vi "Dig a Grave - Complex.vi"() -> ()   [LabVIEW 2017]
doc: "A demonstration of digging graves for slightly more complex legacy code to be refactored. This includes step-by-step instructions for creating grave sin one of two methods: shortcut menu plugin or Quick Drop shortcut plugin. A \"grave\" is a Diagram Disable Structure with a \"Corpse\" disabled frame for the legacy code and a \"Spirit\" enabled frame with a copy of the legacy code to safely refactor."
panel:
  in  "Input":timestamp=timestamp(3614009430.8933406 s since 1904-01-01)
  in  "Stop":bool
  # "Overview: Demonstrates digging a grave for slightly more comple code that needs to be refactored\nInstructions:\n1. Run the VI\n2. Select a time and date using the Input control\n3. Observe the behavior of the VI. Does a notification dialog ever appear?\n4. Switch to the block diagram and follow the instructions there to refactor the code"
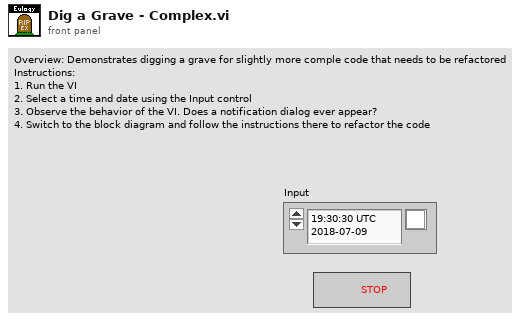
[diagram p1: front panel]
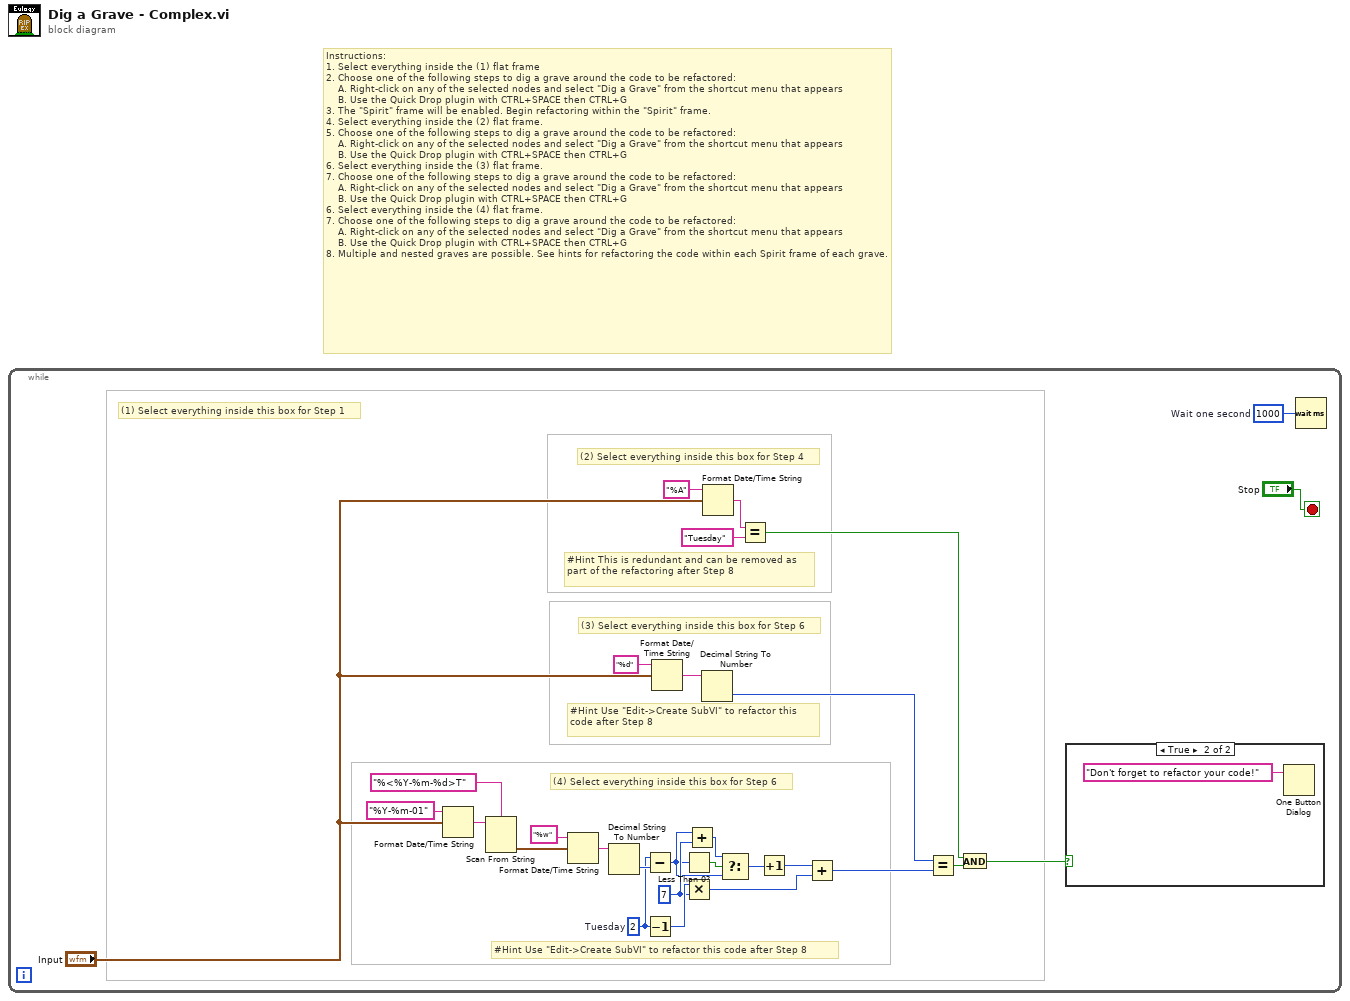
[diagram p0: block diagram]
diagram:
  # "Instructions:\n1. Select everything inside the (1) flat frame\n2. Choose one of the following steps to dig a grave around the code to be refactored:\n    A. Right-click on any of the selected nodes and select \"Dig a Grave\" from the shortcut menu that appears\n    B. Use the Quick Drop plugin with CTRL+SPACE then CTRL+G\n3. The \"Spirit\" frame will be enabled. Begin refactoring within the \"Spirit\" frame.\n4. Select everything inside the (2) flat frame.\n5. Choose one of the following steps to dig a grave around the code to be refactored:\n    A. Right-click on any of the selected nodes and select \"Dig a Grave\" from the shortcut menu that appears\n    B. Use the Quick Drop plugin with CTRL+SPACE then CTRL+G\n6. Select everything inside the (3) flat frame.\n7. Choose one of the following steps to dig a grave around the code to be refactored:\n    A. Right-click on any of the selected nodes and select \"Dig a Grave\" from the shortcut menu that appears\n    B. Use the Quick Drop plugin with CTRL+SPACE then CTRL+G\n6. Select everything inside the (4) flat frame.\n7. Choose one of the following steps to dig a grave around the code to be refactored:\n    A. Right-click on any of the selected nodes and select \"Dig a Grave\" from the shortcut menu that appears\n    B. Use the Quick Drop plugin with CTRL+SPACE then CTRL+G\n8. Multiple and nested graves are possible. See hints for refactoring the code within each Spirit frame of each grave."
  n1 = while {
    stop <- "Stop" stop-if-true
    w13 = 7
    w15 = 2  # Tuesday
    w28 = u32 1000  # Wait one second
    # "#Hint Use \"Edit->Create SubVI\" to refactor this code after Step 8"
    # "(4) Select everything inside this box for Step 6"
    # "#Hint Use \"Edit->Create SubVI\" to refactor this code after Step 8"
    # "#Hint This is redundant and can be removed as part of the refactoring after Step 8"
    # "(3) Select everything inside this box for Step 6"
    # "(2) Select everything inside this box for Step 4"
    # "(1) Select everything inside this box for Step 1"
    n2 = Format Date/Time String(time format string (%c)="%Y-%m-01", seconds (now)="Input") -> (date/time string=w20:string)  [unwired: 1 in]
    n3 = Scan From String(format string="%<%Y-%m-%d>T", input string=w20) -> (output 1=w19:timestamp)  [unwired: 3 in, 3 out]
    n4 = Format Date/Time String(time format string (%c)="%w", seconds (now)=w19) -> (date/time string=w17:string)  [unwired: 1 in]
    n5 = Decimal String To Number(string=w17) -> (number=w16:i32)  [unwired: 2 in, 1 out]
    n6 = Subtract(x=w15, y=w16) -> (x-y=w10:i32)
    n7 = Decrement(x=w15) -> (x-1=w14:i32)
    n8 = Format Date/Time String(time format string (%c)="%d", seconds (now)="Input") -> (date/time string=w25:string)  [unwired: 1 in]
    n9 = Less Than 0?(x=w10) -> (x < 0?=w12:bool)
    n10 = Multiply(x=w14, y=w13) -> (x*y=w7:i32)
    n11 = Add(x=w10, y=w13) -> (x+y=w11:i32)
    n12 = Decimal String To Number(string=w25) -> (number=w4:i32)  [unwired: 2 in, 1 out]
    n13 = Format Date/Time String(time format string (%c)="%A", seconds (now)="Input") -> (date/time string=w24:string)  [unwired: 1 in]
    n14 = Select(t=w11, s=w12, f=w10) -> (s? t:f=w9:i32)
    n15 = Equal?(x=w24, y="Tuesday") -> (x = y?=w6:bool)
    n16 = Increment(x=w9) -> (x+1=w8:i32)
    n17 = Add(x=w8, y=w7) -> (x+y=w5:i32)
    n18 = Equal?(x=w4, y=w5) -> (x = y?=w3:bool)
    n19 = And(x=w6, y=w3) -> (x .and. y?=w2:bool)
    n20 = case shown="True" w2 {
      frame False {
      }
      frame True {
        n21 = One Button Dialog(message="Don't forget to refactor your code!") -> ()  [unwired: 1 in, 1 out]
      }
    }
    n22 = Wait (ms)(milliseconds to wait=w28) -> ()  [unwired: 1 out]
  }
